vi "frontp_generate_UI_user_events.vi"(8 "error in (no error)":errorcluster, 11 "front_panel in":refnum<class "front_panel.lvclass">) -> (0 "error out":errorcluster, 2 "registred_events":T1, 3 "front_panel out":refnum<class "front_panel.lvclass">)   [LabVIEW 2015, in "front_panel.lvclass"]
uses:
  front_panel.lvclass
  ui_registered_events.ctl
  ui_user_events.ctl
  front_panel.lvclass/front_panel.ctl
  panel_class/panel.lvclass
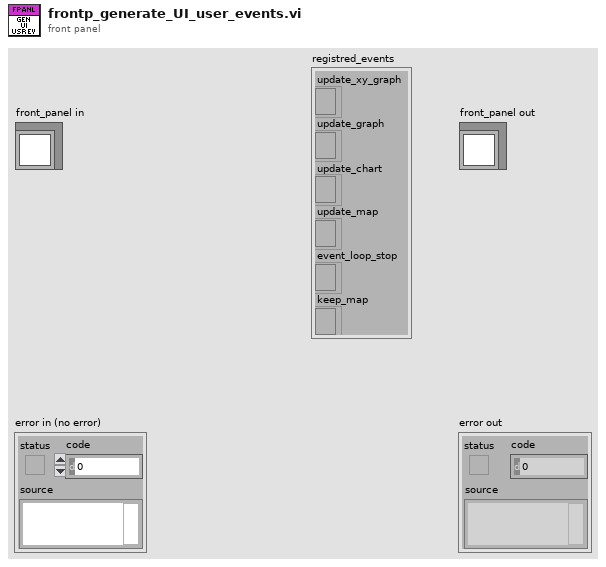
[diagram p1: front panel]
types:
  T1 = typedef "ui_registered_events.ctl" = cluster{"update_xy_graph":refnum<event-registration>, "update_graph":refnum<event-registration>, "update_chart":refnum<event-registration>, "update_map":refnum<event-registration>, "event_loop_stop":refnum<event-registration>, "keep_map":refnum<event-registration>}
  T2 = typedef "ui_user_events.ctl" = cluster{"update_xy_graph":refnum<user-event>, "update_graph":refnum<user-event>, "update_chart":refnum<user-event>, "update_map":refnum<user-event>, "event_loop_stop":refnum<user-event>, "keep_map":refnum<user-event>}
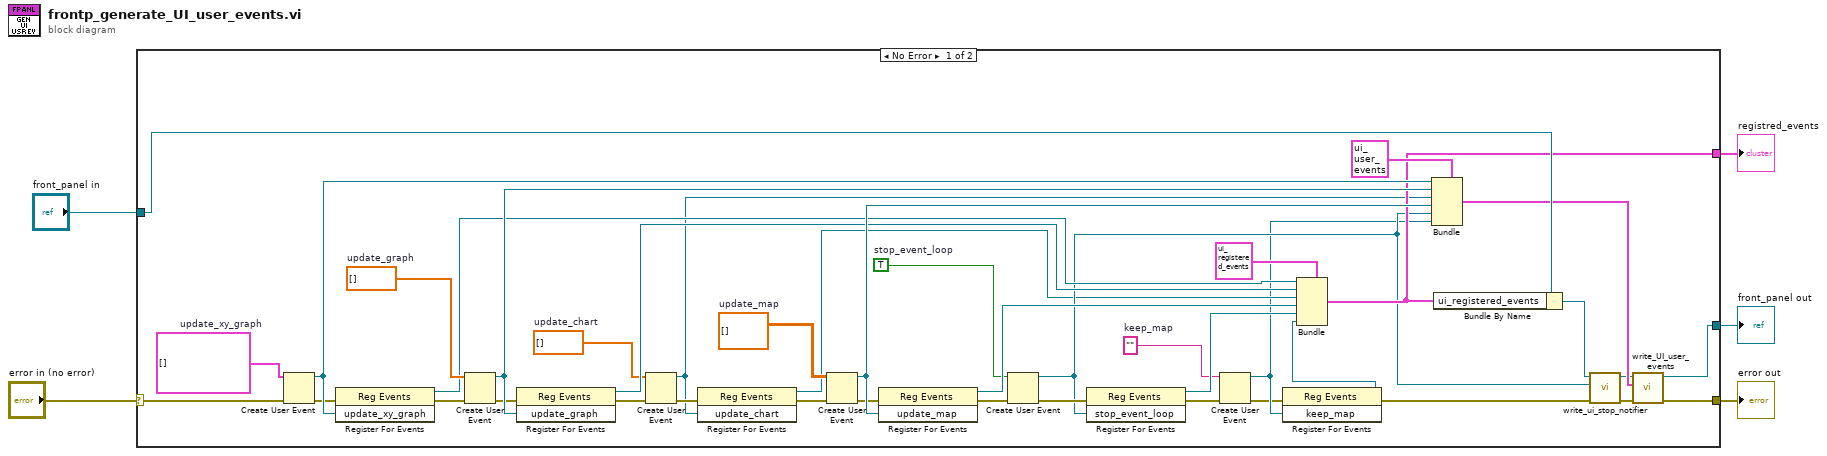
[diagram p0: block diagram]
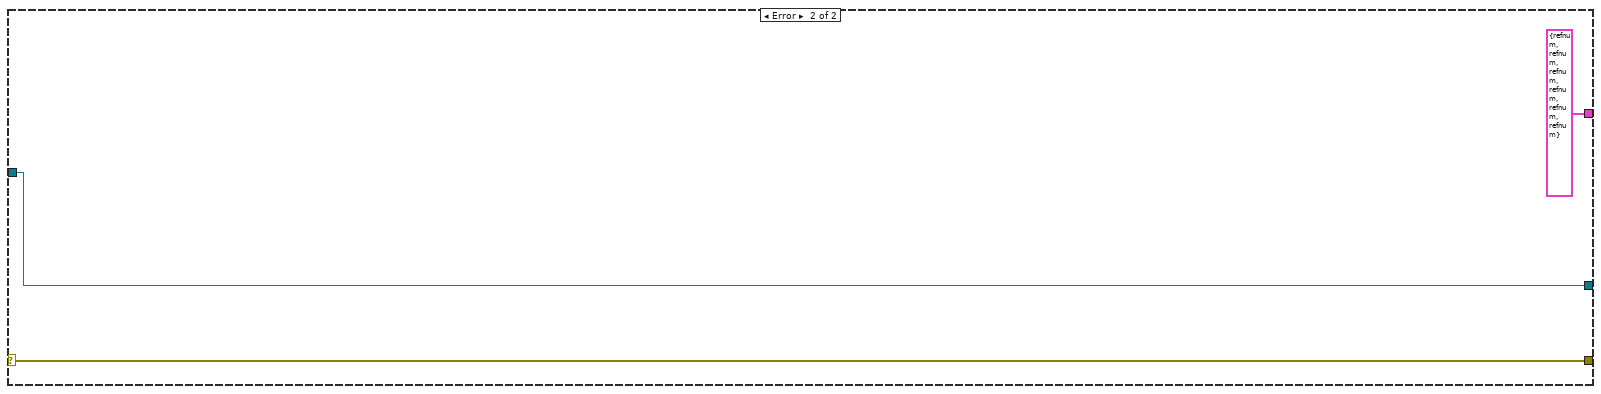
[diagram p2: hidden frame]
diagram:
  n1 = case shown="No Error" "error in (no error)" {
    selector: "error in (no error)" -> [w45 w49]
    tunnel: [w21 w49] -> w4
    tunnel: [w20 w48] -> w2
    tunnel: "front_panel in" -> [w34 w48]
    tunnel: [w26 T1 {"update_xy_graph"=refnum, "update_graph"=refnum, "update_chart"=refnum, "update_map"=refnum, "event_loop_stop"=refnum, "keep_map"=refnum} ("output cluster")] -> w1
    frame No Error {
      w11 = ""  # keep_map
      w14 = dbl[] []  # update_chart
      w24 = TRUE  # stop_event_loop
      w42 = dbl[][] []  # update_map
      w43 = dbl[] []  # update_graph
      w46 = cluster{dbl[], dbl[]}[] []  # update_xy_graph
      n2 = Create User Event(user event datatype=w46, error in=w45) -> (user event=w44:refnum<user-event>, error out=w33:errorcluster)
      n3 = register-events(error in=w33, w44) -> (reference out=w38:refnum<event-registration>, error out=w32:errorcluster)  [unwired: 1 in]
      n4 = Create User Event(user event datatype=w43, error in=w32) -> (user event=w41:refnum<user-event>, error out=w31:errorcluster)
      n5 = register-events(error in=w31, w41) -> (reference out=w37:refnum<event-registration>, error out=w28:errorcluster)  [unwired: 1 in]
      n6 = Create User Event(user event datatype=w14, error in=w28) -> (user event=w13:refnum<user-event>, error out=w27:errorcluster)
      n7 = register-events(error in=w27, w13) -> (reference out=w12:refnum<event-registration>, error out=w30:errorcluster)  [unwired: 1 in]
      n8 = Create User Event(user event datatype=w42, error in=w30) -> (user event=w40:refnum<user-event>, error out=w29:errorcluster)
      n9 = register-events(error in=w29, w40) -> (reference out=w36:refnum<event-registration>, error out=w25:errorcluster)  [unwired: 1 in]
      n10 = Create User Event(user event datatype=w24, error in=w25) -> (user event=w15:refnum<user-event>, error out=w23:errorcluster)
      n11 = register-events(error in=w23, w15) -> (reference out=w22:refnum<event-registration>, error out=w10:errorcluster)  [unwired: 1 in]
      n12 = Create User Event(user event datatype=w11, error in=w10) -> (user event=w9:refnum<user-event>, error out=w8:errorcluster)
      n13 = register-events(error in=w8, w9) -> (reference out=w6:refnum<event-registration>, error out=w7:errorcluster)  [unwired: 1 in]
      n14 = Bundle(cluster=T1 {"update_xy_graph"=refnum, "update_graph"=refnum, "update_chart"=refnum, "update_map"=refnum, "event_loop_stop"=refnum, "keep_map"=refnum} ("output cluster"), "update_xy_graph"=w38, "update_graph"=w37, "update_chart"=w12, "update_map"=w36, "event_loop_stop"=w22, "keep_map"=w6) -> (w26:T1)
      n15 = Bundle(cluster=T2 {"update_xy_graph"=refnum, "update_graph"=refnum, "update_chart"=refnum, "update_map"=refnum, "event_loop_stop"=refnum, "keep_map"=refnum} ("output cluster"), "update_xy_graph"=w44, "update_graph"=w41, "update_chart"=w13, "update_map"=w40, "event_loop_stop"=w15, "keep_map"=w9) -> (w19:T2)
      n16 = Bundle By Name(cluster=w34, "ui_registered_events"=w26) -> (w17:refnum<class "front_panel.lvclass">)
      n17 = call "write_ui_stop_notifier.vi"("error in (no error)"=w7, "stop_ui_notifier"=w15, "panel in"=w17) -> ("error out"=w18:errorcluster, "panel out"=w16:refnum<class "front_panel.lvclass">)  [unwired: 7 in]
      n18 = call "write_UI_user_events.vi"("error in (no error)"=w18, "ui_events"=w19, "panel in"=w16) -> ("error out"=w21:errorcluster, "panel out"=w20:refnum<class "front_panel.lvclass">)  [unwired: 7 in]
    }
    frame Error {
    }
  }
  "error out" <- w4
  "front_panel out" <- w2
  "registred_events" <- w1
